vi "get_indexArray.vi"(0 "HGF_FGV_SelectByName":refnum<class "HGF_FGV_SelectByName.lvclass">, 5 "error in (no error)":errorcluster) -> (14 "dup HGF_FGV_SelectByName":refnum<class "HGF_FGV_SelectByName.lvclass">, 16 "indexArray":u32[](array[numeric]), 19 "error out":errorcluster)   [LabVIEW 2012, in "HGF_FGV.lvlib" / "HGF_FGV_SelectByName.lvclass"]
doc: "Returns index array of addressed objects."
uses:
  HGF_FGV_SelectByName.lvclass
  HGF_FGV_SelectByName.lvclass/HGF_FGV_SelectByName.ctl
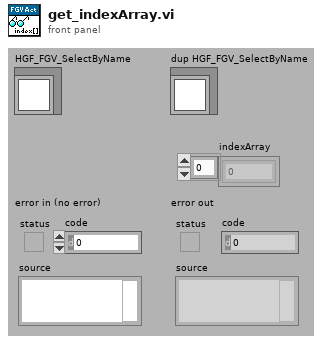
[diagram p1: front panel]
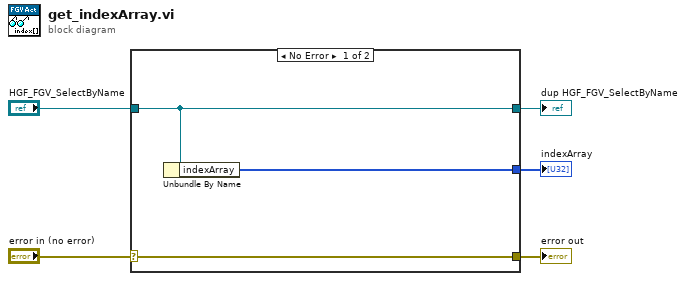
[diagram p0: block diagram]
diagram:
  n1 = case shown="No Error" "error in (no error)" {
    selector: "error in (no error)" -> [w8 w9]
    tunnel: [w8 w9] -> w4
    tunnel: [w7 w10] -> w2
    tunnel: "HGF_FGV_SelectByName" -> [w7 w10]
    tunnel: [w6 _] -> w1
    frame No Error {
      n2 = Unbundle By Name(w7) -> ("indexArray"=w6:u32[])
    }
    frame Error {
    }
  }
  "error out" <- w4
  "dup HGF_FGV_SelectByName" <- w2
  "indexArray" <- w1
